vi "EIP Single Channel.vi"(8 "error in (no error)":errorcluster, 11 "Node Ptr":T2 format="%.0x") -> (0 "error out":errorcluster)   [LabVIEW 2011, in "Ethernet IP Custom Device Custom Device.lvlib"]
uses:
  Ethernet IP Custom Device Custom Device.lvlib
  <vilib>/NI Veristand/Custom Device API/Custom Device Item Ref.ctl
  L5K Data Types.ctl
  Ethernet IP Global Strings.vi
  <vilib>/NI Veristand/Custom Device API/Get Item Property (U16).vi
  <vilib>/NI Veristand/Custom Device API/Get Item Property (String).vi
  <vilib>/NI Veristand/Custom Device API/Custom Device API.lvlib
panel:
  in  "Default Value":dbl
  out "Data Type":T1
  in  "Description":string
  out "Tag Name":string
  in  "Header":cluster{"Section Name":string}={"Section Name"="Custom Device Item Settings"}
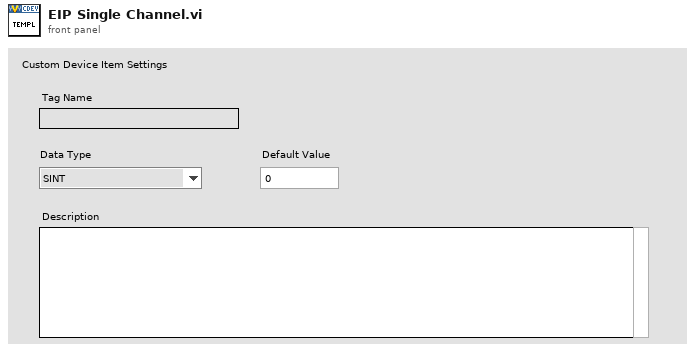
[diagram p1: front panel]
types:
  T1 = typedef "Ethernet IP Custom Device Custom Device.lvlib/L5K Data Types.ctl" = enum16{"SINT", "INT", "DINT", "REAL", "BOOL"}
  T2 = typedef "Custom Device API.lvlib/Custom Device Item Ref.ctl" = u64
  T3 = typedef "Custom Device API.lvlib/Custom Device Channel.ctl" = cluster{"Type":T4, "Units":string, "Default Value":dbl, "Faultable":bool, "Scalable":bool}
  T4 = typedef "Custom Device API.lvlib/Custom Device Channel Type.ctl" = enum16{"Input", "Output"}
  T5 = typedef "Custom Device API.lvlib/Custom Device Commands.ctl" = enum16{"Default", "Item renamed", "Shutdown", "Dynamic button pressed"}
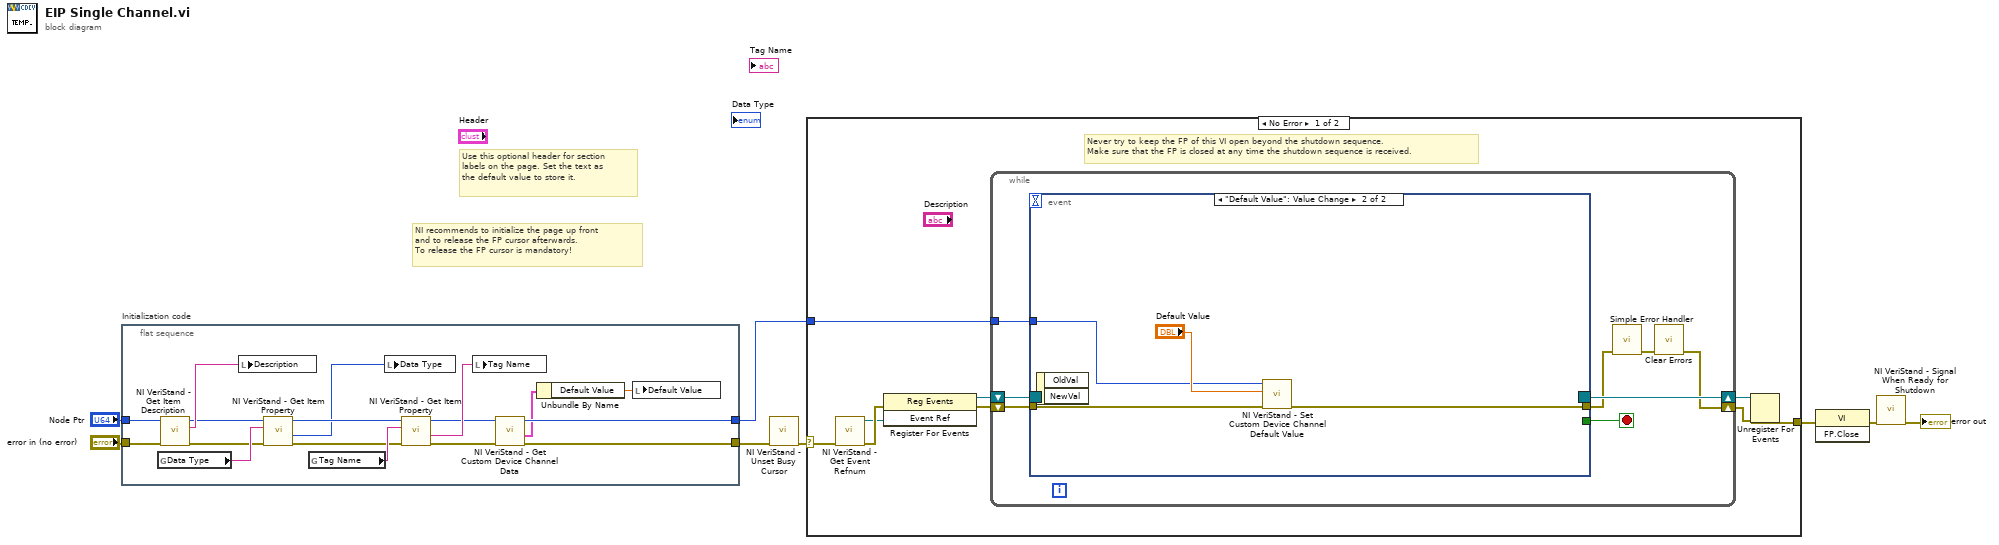
[diagram p0: block diagram]
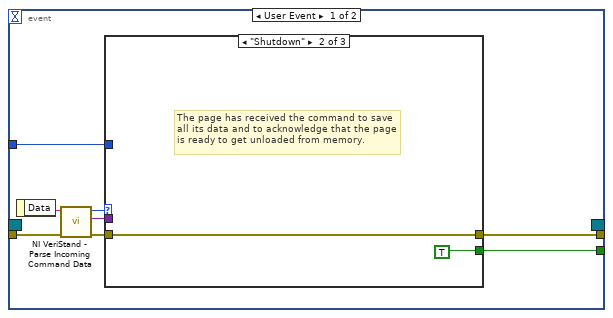
[diagram p2: hidden frame]
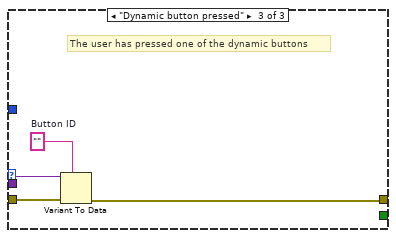
[diagram p4: hidden frame]
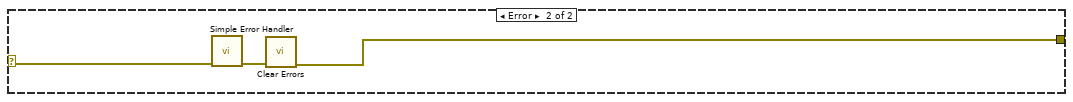
[diagram p5: hidden frame]
diagram:
  # "Use this optional header for section labels on the page. Set the text as the default value to store it."
  # "NI recommends to initialize the page up front\nand to release the FP cursor afterwards.\nTo release the FP cursor is mandatory!"
  n1 = flat-sequence "Initialization code" {
    tunnel: "error in (no error)" -> [w25]
    tunnel: "Node Ptr" -> [w24]
    tunnel: [w11] -> w4
    tunnel: [w12] -> w1
    frame #0 {
      n2 = global read "Ethernet IP Global Strings.vi" "Data Type"() -> (w20:string)
      n3 = call <vilib>:"NI VeriStand - Get Item Description.vi"("error in (no error)"=w25, "Item Ref in"=w24) -> ("error out"=w18:errorcluster, "Description"=w23:string, "Item Ref out"=w22:T2)  [unwired: 7 out]
      n4 = local write "Description"(w23) -> ()
      n5 = call-poly <vilib>:"NI VeriStand - Get Item Property.vi"("error in (no error)"=w18, "Property Name"=w20, "Item Ref in"=w22) -> ("error out"=w17:errorcluster, "Value"=w16:u16, "Item Ref out"=w21:T2)  [unwired: 5 in, 1 out]
      n6 = global read "Ethernet IP Global Strings.vi" "Tag Name"() -> (w19:string)
      n7 = local write "Data Type"(w16) -> ()
      n8 = call-poly <vilib>:"NI VeriStand - Get Item Property.vi"("error in (no error)"=w17, "Property Name"=w19, "Item Ref in"=w21) -> ("error out"=w14:errorcluster, "Value"=w15:string, "Item Ref out"=w13:T2)  [unwired: 5 in, 1 out]
      n9 = local write "Tag Name"(w15) -> ()
      n10 = call <vilib>:"NI VeriStand - Get Custom Device Channel Data.vi"("error in (no error)"=w14, "Channel Ref in"=w13) -> ("error out"=w11:errorcluster, "Channel"=w10:T3, "Channel Ref out"=w12:T2)  [unwired: 4 in, 3 out]
      n11 = Unbundle By Name(w10) -> ("Default Value"=w9:dbl)
      n12 = local write "Default Value"(w9) -> ()
    }
  }
  n13 = call <vilib>:"NI VeriStand - Unset Busy Cursor.vi"("error in (no error)"=w4) -> ("error out"=w3:errorcluster)  [unwired: 10 out]
  n14 = case shown="No Error" w3 {
    selector: w3 -> [w26 w64]
    tunnel: [w31 w62] -> w8
    tunnel: w1 -> [w27 _]
    frame No Error {
      # "Never try to keep the FP of this VI open beyond the shutdown sequence.\nMake sure that the FP is closed at any time the shutdown sequence is received."
      n15 = call <vilib>:"NI VeriStand - Get Event Refnum.vi"("error in (no error)"=w26) -> ("error out"=w34:errorcluster, "Event Ref"=w30:refnum<user-event>)  [unwired: 9 out]
      n16 = register-events(error in=w34, w30) -> (reference out=w28:refnum<event-registration>, error out=w29:errorcluster)  [unwired: 1 in]
      n17 = while {
        tunnel: w27 -> [w38]
        shift-right: [w35] -> w32
        shift-left: w29 -> [w41]
        shift-right: [w42] -> w33
        shift-left: w28 -> [w40]
        stop <- w39 stop-if-true
        n18 = event shown="[1] \"Default Value\": Value Change" {
          selector: w40 -> [_ _]
          dyn-events: [_ _] -> w42
          timeout: _ -> [_ _]
          tunnel: w41 -> [w50 w61]
          tunnel: [w46 _] -> w39
          tunnel: [w45 w58] -> w37
          tunnel: w38 -> [w44 w59]
          event User Event {
            n19 = event-data() -> ("Data"=w49:string)  [unwired: 1 out]
            n20 = call <vilib>:"NI VeriStand - Parse Incoming Command Data.vi"("error in (no error)"=w50, "Incoming data"=w49) -> ("error out"=w48:errorcluster, "Outgoing data"=w43:variant, "Action"=w47:T5)  [unwired: 7 out]
            n21 = case shown="\"Shutdown\"" w47 {
              tunnel: w48 -> [w51 w52 w57]
              tunnel: [_ TRUE _] -> w46
              tunnel: [w51 w52 w54] -> w45
              tunnel: w44 -> [_ _ _]
              tunnel: w43 -> [_ _ w56]
              frame "Default", Default {
              }
              frame "Shutdown" {
                # "The page has received the command to save all its data and to acknowledge that the page is ready to get unloaded from memory."
              }
              frame "Dynamic button pressed" {
                w55 = ""  # Button ID
                # "The user has pressed one of the dynamic buttons"
                n22 = Variant To Data(error in=w57, type=w55, Variant=w56) -> (error out=w54:errorcluster)  [unwired: 1 out]
              }
            }
          }
          event "Default Value": Value Change {
            n23 = event-data() -> ()  [unwired: 3 out]
            n24 = call <vilib>:"NI VeriStand - Set Custom Device Channel Default Value.vi"("error in (no error)"=w61, "Default Value"="Default Value", "Channel Ref in"=w59) -> ("error out"=w58:errorcluster)  [unwired: 7 in, 1 out]
          }
        }
        n25 = call <vilib>:"Simple Error Handler.vi"("error in (no error)"=w37) -> ("error out"=w36:errorcluster)  [unwired: 1 in, 7 out]
        n26 = call <vilib>:"Clear Errors.vi"("error in (no error)"=w36) -> ("error out"=w35:errorcluster)  [unwired: 6 out]
      }
      n27 = Unregister For Events(event registration refnum=w33, error in=w32) -> (error out=w31:errorcluster)
    }
    frame Error {
      n28 = call <vilib>:"Simple Error Handler.vi"("error in (no error)"=w64) -> ("error out"=w63:errorcluster)  [unwired: 1 in, 7 out]
      n29 = call <vilib>:"Clear Errors.vi"("error in (no error)"=w63) -> ("error out"=w62:errorcluster)  [unwired: 6 out]
    }
  }
  n30 = invoke class="VI" method="FP.Close"(error in=w8) -> (error out=w7:errorcluster)  [unwired: 2 in, 2 out]
  n31 = call <vilib>:"NI VeriStand - Signal When Ready for Shutdown.vi"("error in (no error)"=w7) -> ("error out"=→"error out":errorcluster)  [unwired: 10 out]
